vi "Set Variant.vi"(0 "image in":refnum<class "MSC Image.lvclass">, 1 "Variant":variant, 5 "error in (no error)":errorcluster) -> (14 "image out":refnum<class "MSC Image.lvclass">, 19 "error out":errorcluster)   [LabVIEW 2014, in "MSC Image.lvclass"]
doc: "Sets the image variant. Use this for e.g. comments, parameters or references."
uses:
  MSC Image.lvclass
  MSC Image.lvclass/MSC Image.ctl
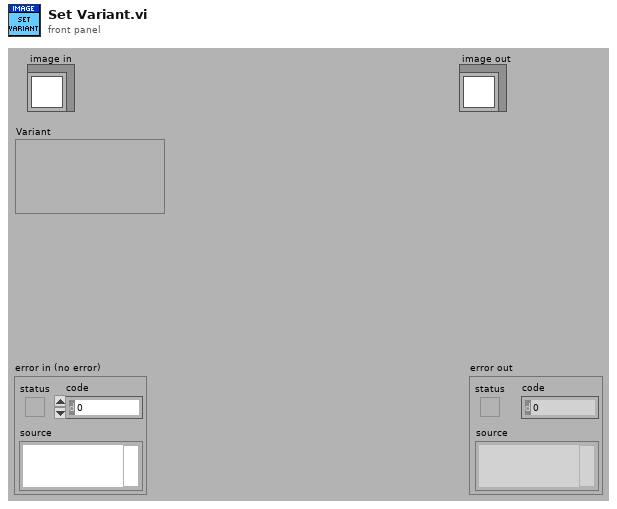
[diagram p1: front panel]
types:
  T1 = typedef "Image.ctl" = cluster{"Pointer":u64, "Size":T2, "Image Type":T3, "Time Stamp":timestamp, "Variant":variant}
  T2 = typedef "Size.ctl" = cluster{"Cols":i32, "Rows":i32}
  T3 = typedef "Image Type.ctl" = i32
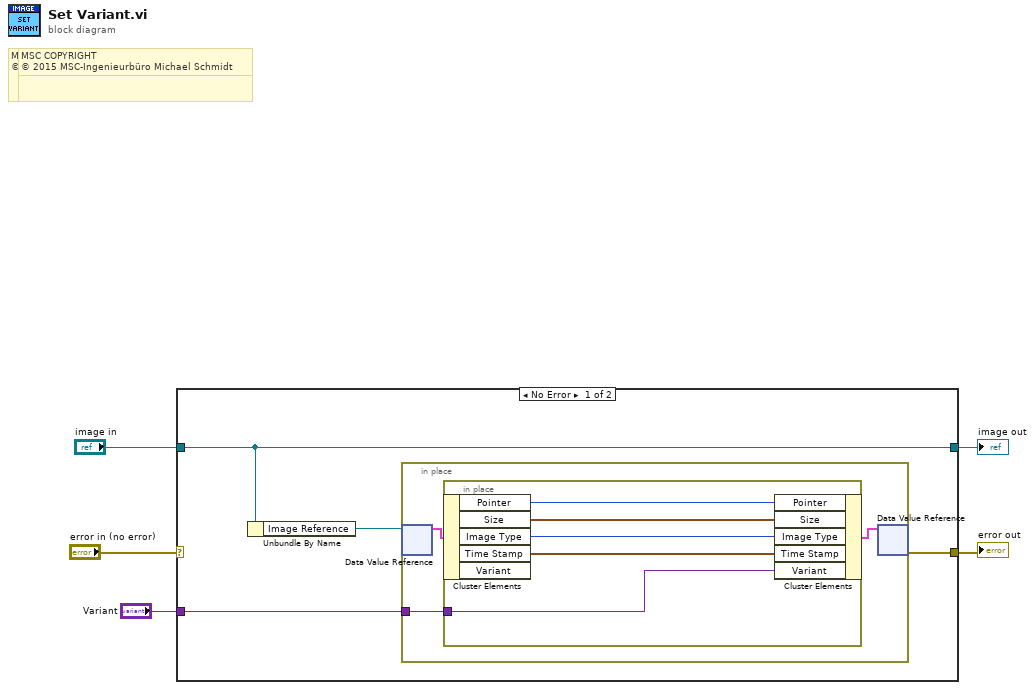
[diagram p0: block diagram]
diagram:
  # "MSC COPYRIGHT\n© 2016 MSC-Ingenieurbüro Michael Schmidt"
  # "MSC COPYRIGHT\n© 2016 MSC-Ingenieurbüro Michael Schmidt"
  # "MSC COPYRIGHT\n© 2015 MSC-Ingenieurbüro Michael Schmidt"
  # "MSC COPYRIGHT\n© 2015 MSC-Ingenieurbüro Michael Schmidt"
  n1 = case shown="No Error" "error in (no error)" {
    selector: "error in (no error)" -> [_ w19]
    tunnel: [w7 w19] -> w4
    tunnel: [w9 w18] -> w2
    tunnel: "image in" -> [w9 w18]
    tunnel: "Variant" -> [w6 _]
    frame No Error {
      n2 = Unbundle By Name(w9) -> ("Image Reference"=w8:refnum<data-value>)
      n3 = in-place {
        in-place-border: w6 -> [w10]
        n4 = in-place-dvr #1(w8) -> (w11:T1)  [unwired: 1 out]
        n5 = in-place {
          in-place-border: w10 -> [w13]
          n6 = in-place-cluster #2(w11) -> ("Pointer"=w17:u64, "Size"=w14:T2, "Image Type"=w16:T3, "Time Stamp"=w15:timestamp)  [unwired: 1 out]
          n7 = in-place-cluster #2("Pointer"=w17, "Size"=w14, "Image Type"=w16, "Time Stamp"=w15, "Variant"=w13) -> (w12:T1)
        }
        n8 = in-place-dvr #1(w12) -> (w7:errorcluster)  [unwired: 1 out]
      }
    }
    frame Error {
    }
  }
  "error out" <- w4
  "image out" <- w2
